vi "Run_EnFlo_Hub.vi"(4 "Error In":errorcluster) -> (0 "Error Out":errorcluster)   [LabVIEW 2015]
uses:
  Anemometry Sub Vis/Globals/Dynamic_call_global.ph.vi
panel:
  out "No of iterations":i32
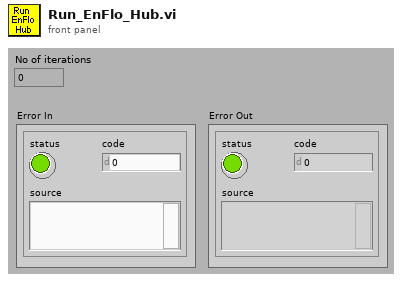
[diagram p1: front panel]
types:
  T1 = enum32{"Bad", "Idle", "Run top level", "Running"}
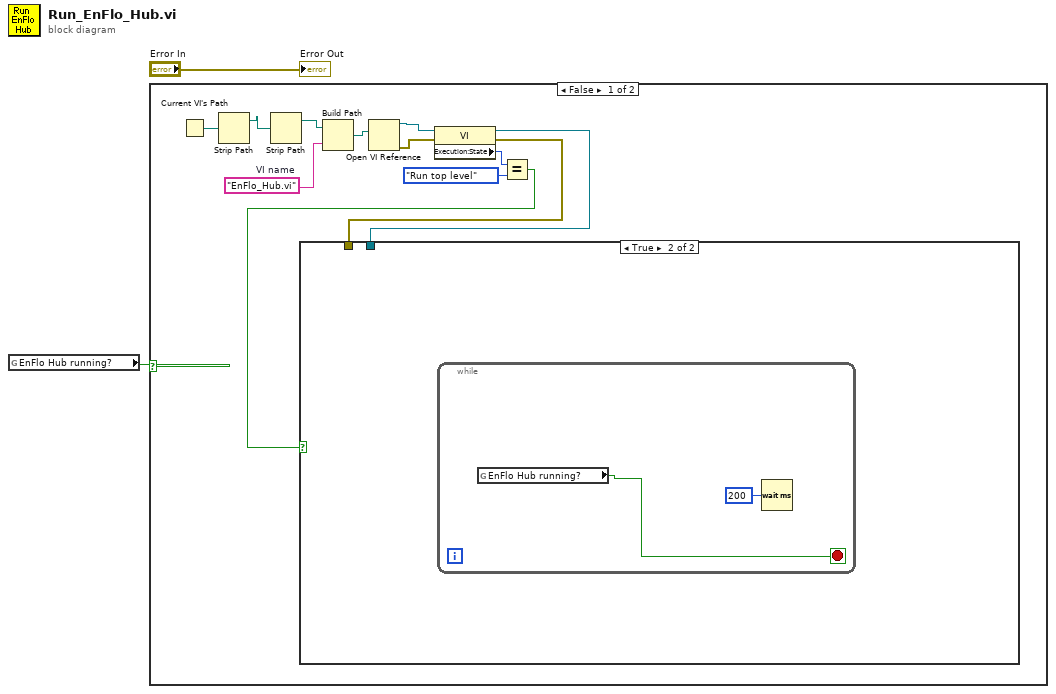
[diagram p0: block diagram]
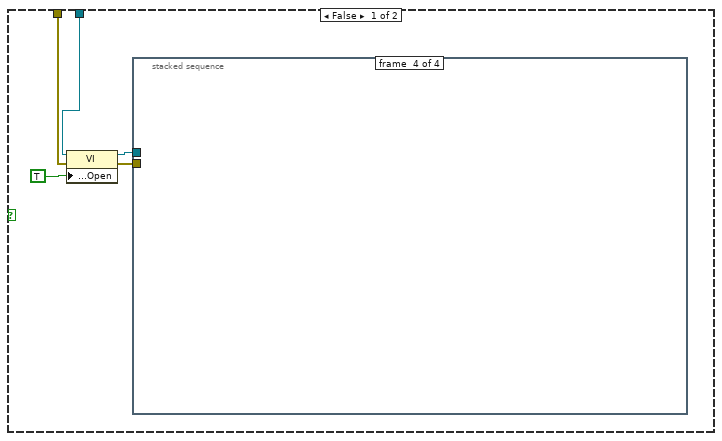
[diagram p2: hidden frame]
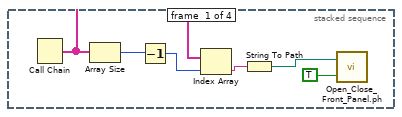
[diagram p3: hidden frame]
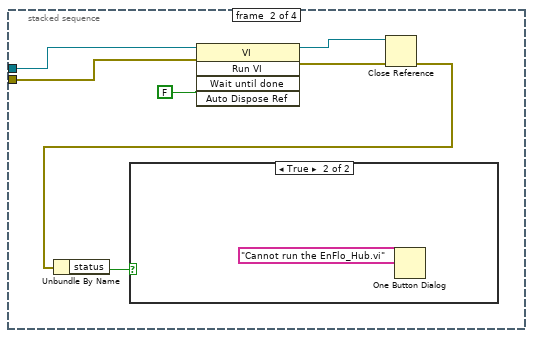
[diagram p4: hidden frame]
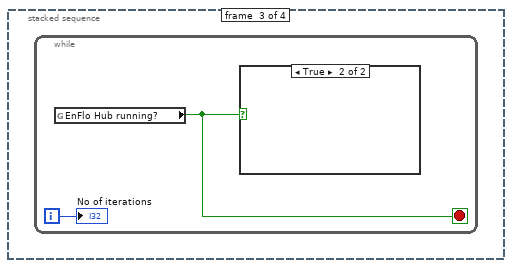
[diagram p6: hidden frame]
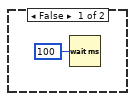
[diagram p7: hidden frame]
diagram:
  n1 = global read "Dynamic_call_global.ph.vi" "EnFlo Hub running?"() -> (w2:bool)
  n2 = case shown="False" w2 {
    frame False {
      w9 = "EnFlo_Hub.vi"  # VI name
      n3 = Current VI's Path() -> (path=w8:path)
      n4 = Strip Path(path=w8) -> (stripped path=w10:path)  [unwired: 1 out]
      n5 = Strip Path(path=w10) -> (stripped path=w11:path)  [unwired: 1 out]
      n6 = Build Path(base path=w11, name or relative path=w9) -> (appended path=w14:path)
      n7 = Open VI Reference(vi path=w14) -> (vi reference=w12:refnum<vi>, error out=w13:errorcluster)  [unwired: 2 in, 3 out]
      n8 = property class="VI"(reference=w12, error in=w13) -> (reference out=w3:refnum<vi>, error out=w4:errorcluster, "Execution:State"=w7:T1)
      n9 = Equal?(x=w7, y=T1."Run top level" ("Execution:State")) -> (x = y?=w5:bool)
      n10 = case shown="True" w5 {
        tunnel: w4 -> [w18 _]
        tunnel: w3 -> [w17 _]
        frame False {
          n11 = property class="VI"(reference=w17, error in=w18, "Front Panel Window:Open"=TRUE) -> (reference out=w16:refnum<vi>, error out=w15:errorcluster)
          n12 = stacked-sequence {
            tunnel: w16 -> [_ w27 _ _]
            tunnel: w15 -> [_ w26 _ _]
            frame #0 {
              n13 = Call Chain() -> (call chain=w20:string[])
              n14 = Array Size(array=w20) -> (size(s)=w25:i32)
              n15 = Decrement(x=w25) -> (x-1=w24:i32)
              n16 = Index Array(array=w20, index=w24) -> (element=w23:string)
              n17 = String To Path(string=w23) -> (path=w22:path)
              n18 = call "Open_Close_Front_Panel.ph.vi"("Front Panel Window:Open"=TRUE, "VI path"=w22) -> ()  [unwired: 2 out]
            }
            frame #1 {
              w32 = FALSE ("Wait until done")
              n19 = invoke class="VI" method="Run VI"(reference=w27, error in=w26, "Wait until done"=w32, "Auto Dispose Ref"=w32) -> (reference out=w31:refnum<vi>, error out=w30:errorcluster)  [unwired: 1 in, 3 out]
              n20 = Close Reference(reference=w31, error in (no error)=w30) -> (error out=w29:errorcluster)
              n21 = Unbundle By Name(w29) -> ("status"=w28:bool)
              n22 = case shown="True" w28 {
                frame False {
                }
                frame True {
                  n23 = One Button Dialog(message="Cannot run the EnFlo_Hub.vi") -> ()  [unwired: 2 out]
                }
              }
            }
            frame #2 {
              n24 = while {
                i -> [w34]
                stop <- w35 stop-if-true
                n25 = global read "Dynamic_call_global.ph.vi" "EnFlo Hub running?"() -> (w35:bool)
                n26 = case shown="True" w35 {
                  frame False {
                    n27 = Wait (ms)(milliseconds to wait=u32 100) -> ()  [unwired: 1 out]
                  }
                  frame True {
                  }
                }
                "No of iterations" <- w34
              }
            }
            frame #3 {
            }
          }
        }
        frame True {
          n28 = while {
            stop <- w38 stop-if-true
            n29 = global read "Dynamic_call_global.ph.vi" "EnFlo Hub running?"() -> (w38:bool)
            n30 = Wait (ms)(milliseconds to wait=u32 200) -> ()  [unwired: 1 out]
          }
        }
      }
    }
    frame True {
    }
  }
  "Error Out" <- "Error In"
